vi "String 2 Path memory.vi"(0 "Input String":string, 1 "Clear Memory":bool) -> (2 "path":path)   [LabVIEW 2022 SP3]
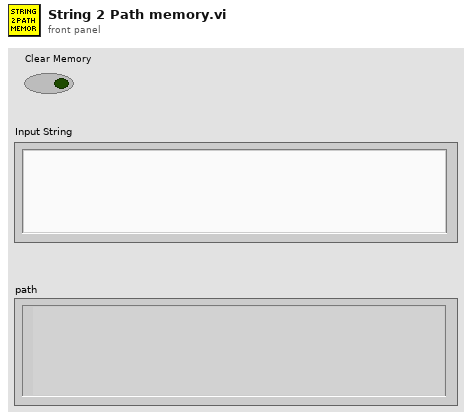
[diagram p1: front panel]
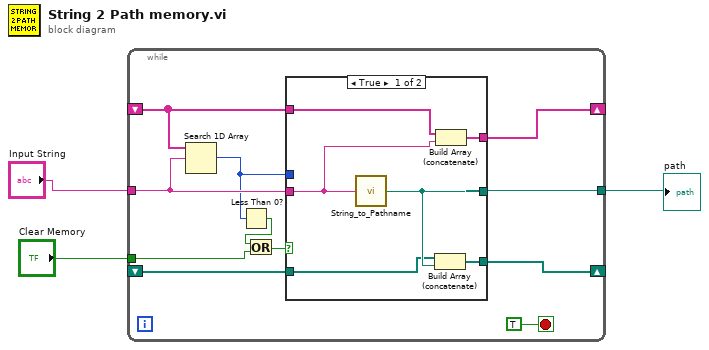
[diagram p0: block diagram]
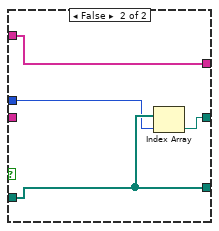
[diagram p2: hidden frame]
diagram:
  n1 = while {
    tunnel: [w14] -> w3
    tunnel: "Input String" -> [w13]
    shift-right: [w11] -> _
    shift-left: _ -> [w12]
    shift-right: [w9] -> _
    shift-left: _ -> [w10]
    tunnel: "Clear Memory" -> [w5]
    stop <- TRUE stop-if-true
    n2 = Search 1D Array(1D array=w12, element=w13) -> (index of element=w4:i32)  [unwired: 1 in]
    n3 = Less Than 0?(x=w4) -> (x < 0?=w6:bool)
    n4 = Or(x=w6, y=w5) -> (x .or. y?=w7:bool)
    n5 = case shown="True" w7 {
      tunnel: [w17 w22] -> w14
      tunnel: w13 -> [w20 _]
      tunnel: w12 -> [w19 w24]
      tunnel: [w18 w24] -> w11
      tunnel: w10 -> [w16 w23]
      tunnel: [w15 w23] -> w9
      tunnel: w4 -> [_ w21]
      frame True {
        n6 = call "String_to_Pathname.vi"("Input String"=w20) -> ("path"=w17:path)
        n7 = Build Array (concatenate)(w16, w17) -> (w15:path[])
        n8 = Build Array (concatenate)(w19, w20) -> (w18:string[])
      }
      frame False {
        n9 = Index Array(array=w23, index=w21) -> (element=w22:path)
      }
    }
  }
  "path" <- w3
